vi "Main_002.vi"() -> ()   [LabVIEW 2025]
uses:
  Utility/Universal Utility/TypeDefs_Utility/Cluster_Row-Column.ctl
  9e3f57c0-2ef8-4495-8287-c6a42a5fb955.vi
  Utility/Universal Utility/TypeDefs_Utility/ENUM_4 Directions U-D-L-R.ctl
  Utility/Universal Utility/TypeDefs_Utility/ENUM_8 Directions U-D-L-R.ctl
panel:
  out "MAX U64":u64
  out "Array":u64[](array[numeric])
  out "MATCH":bool
  in  "Select Data":enum32{"Example", "Puzzle"}(tab)
  in  "Max Number":u64=90
  in  "EX Target":u64=44
  in  "Puzzle  Max Number":u64=4000000
  in  "Puzzle Target":u64=4613732
  out "Answer":u64
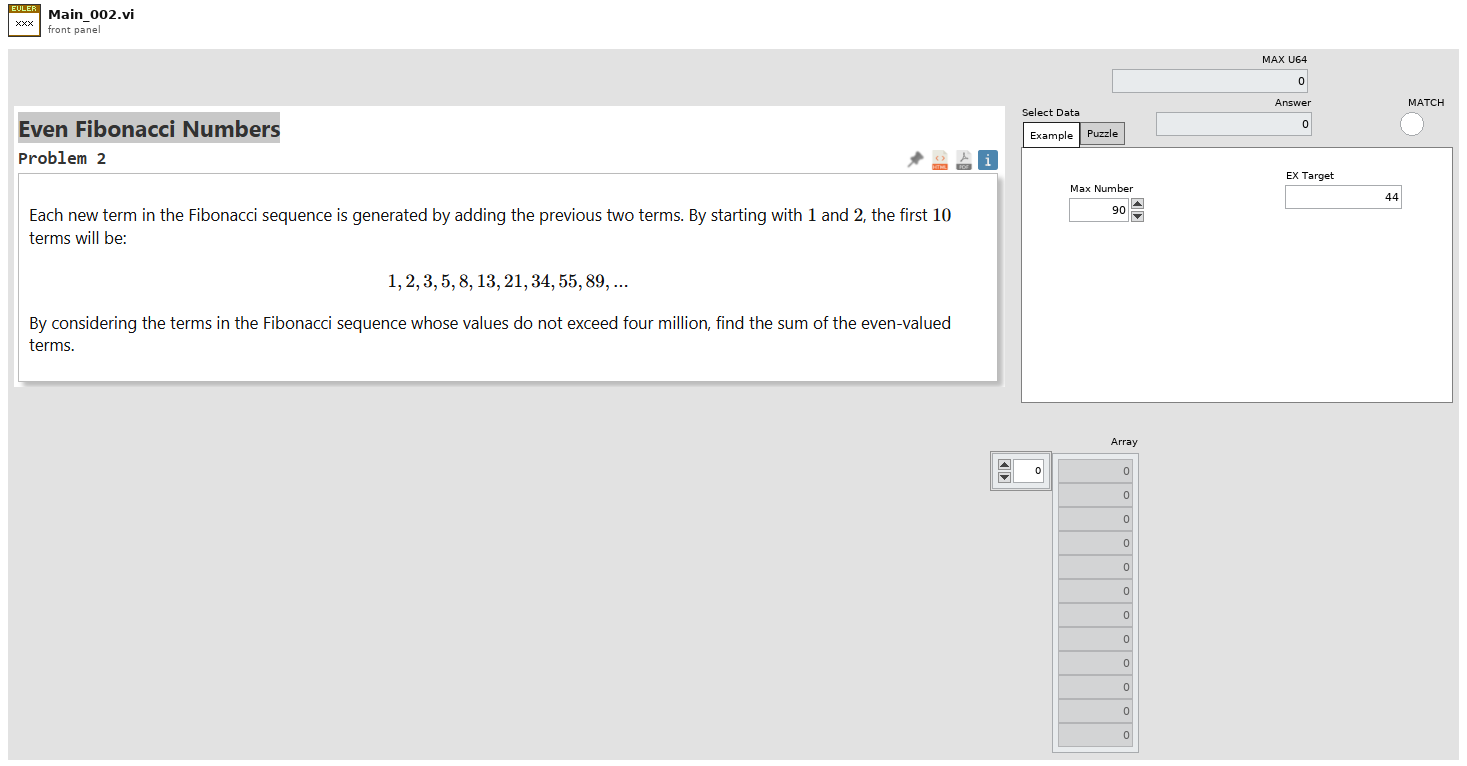
[diagram p1: front panel]
types:
  T1 = typedef "ENUM_8 Directions U-D-L-R.ctl" = enum16{"Up;-1,0", "Up-Right;-1,1", "Right;0,1", "Down-Right;1,1", "Down;1,0", "Down-Left;1,-1", "Left;0,-1", "Up-Left;-1,-1"}
  T2 = typedef "ENUM_4 Directions U-D-L-R.ctl" = enum16{"Up;-1,0", "Right;0,1", "Down;1,0", "Left;0,-1"}
  T3 = typedef "Cluster_Row-Column.ctl" = cluster{"R":i32, "C":i32}
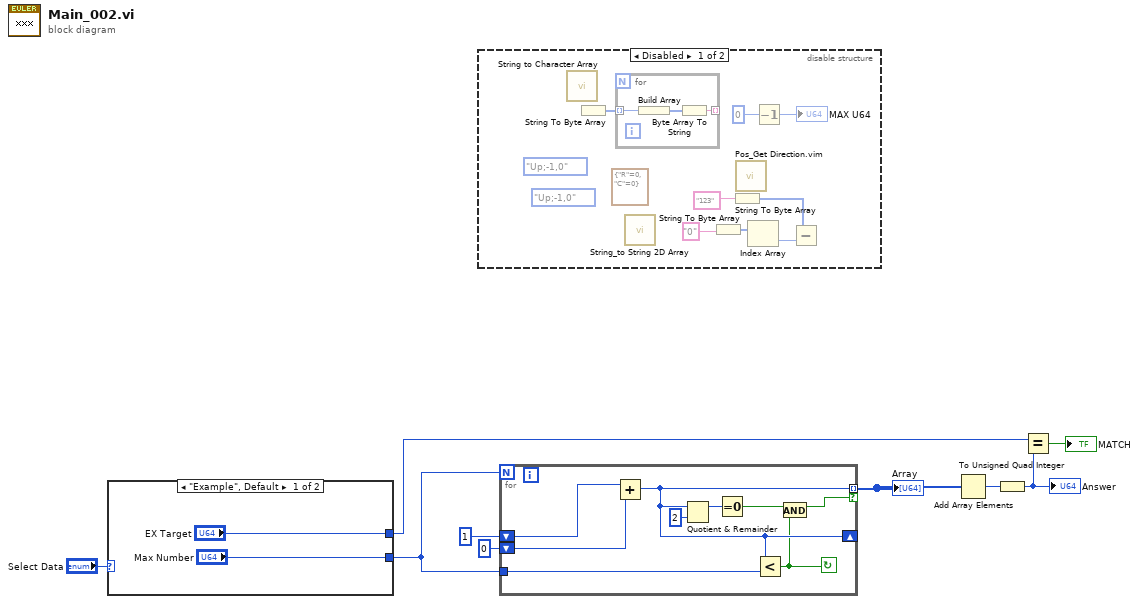
[diagram p0: block diagram]
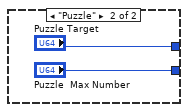
[diagram p2: hidden frame]
diagram:
  n1 = case shown="\"Example\", Default" "Select Data" {
    tunnel: ["Max Number" "Puzzle  Max Number"] -> w1
    tunnel: ["EX Target" "Puzzle Target"] -> w7
    frame "Example", Default {
    }
    frame "Puzzle" {
    }
  }
  n2 = disable-structure shown="Disabled" {
    frame Disabled {
      (unwired) ENUM_8_Directions_U-D-L-R."Up;-1,0" ("Direction 8")
      (unwired) ENUM_4_Directions_U-D-L-R."Up;-1,0" ("Direction")
      (unwired) T3 {"R"=0, "C"=0} ("Position")
      n3 = call "String to Character Array.vi"() -> ()  [unwired: 1 in, 1 out]
      n4 = String To Byte Array() -> (unsigned byte array=w16:u8[])  [unwired: 1 in]
      n5 = for {
        tunnel: w16 -> [w24] mode=indexing
        tunnel: [w22] -> _ mode=indexing
        n6 = Build Array(w24) -> (w23:u8[])
        n7 = Byte Array To String(unsigned byte array=w23) -> (string=w22:string)
      }
      n8 = call "String_to String 2D Array.vi"() -> ()  [unwired: 11 in, 1 out]
      n9 = String To Byte Array(string="0") -> (unsigned byte array=w19:u8[])
      n10 = String To Byte Array(string="123") -> (unsigned byte array=w17:u8[])
      n11 = call "Pos_Get Direction.vim"() -> ()  [unwired: 11 in, 1 out]
      n12 = Index Array(array=w19) -> (element=w18:u8)  [unwired: 1 in]
      n13 = Decrement(x=u64 0 ("sum")) -> (x-1=→"MAX U64":u64)
      n14 = Subtract(x=w17, y=w18) -> ()  [unwired: 1 out]
    }
    frame Enabled {
    }
  }
  n15 = for {
    N: w1 -> [_]
    tunnel: [w27] -> w3 mode=indexing if=w28
    shift-right: [w27] -> _
    shift-left: u64 1 ("x+y") -> [w33]
    shift-left: u64 0 ("x+y") -> [w32]
    tunnel: w1 -> [w26]
    stop <- w25 continue-if-true
    n16 = Add(x=w33, y=w32) -> (x+y=w27:u64)
    n17 = Quotient & Remainder(x=w27, y=u64 2) -> (x-y*floor(x/y)=w30:u64)  [unwired: 1 out]
    n18 = Equal To 0?(x=w30) -> (x = 0?=w29:bool)
    n19 = Less?(x=w27, y=w26) -> (x < y?=w25:bool)
    n20 = And(x=w29, y=w25) -> (x .and. y?=w28:bool)
  }
  "Array" <- w3
  n21 = Add Array Elements(numeric array=w3) -> (sum=w2:u64)
  n22 = To Unsigned Quad Integer(1:w2) -> (0:w6:u64)
  "Answer" <- w6
  n23 = Equal?(x=w7, y=w6) -> (x = y?=→"MATCH":bool)
